vi "thorlabs_set_loopiness.vi"(8 "error in (no error)":errorcluster, 9 "PositionControlMode":i16, 10 "channel":i16, 11 "thorlabs_kinesis in":refnum<class "thorlabs_kinesis.lvclass">) -> (0 "error out":errorcluster, 3 "thorlabs_kinesis out":refnum<class "thorlabs_kinesis.lvclass">)   [LabVIEW 2015, in "thorlabs_kinesis.lvclass"]
uses:
  thorlabs_kinesis.lvclass
  thorlabs_kinesis.lvclass/thorlabs_kinesis.ctl
  thorlabs_drivers/Thorlabs.MotionControl.Benchtop.Piezo.dll
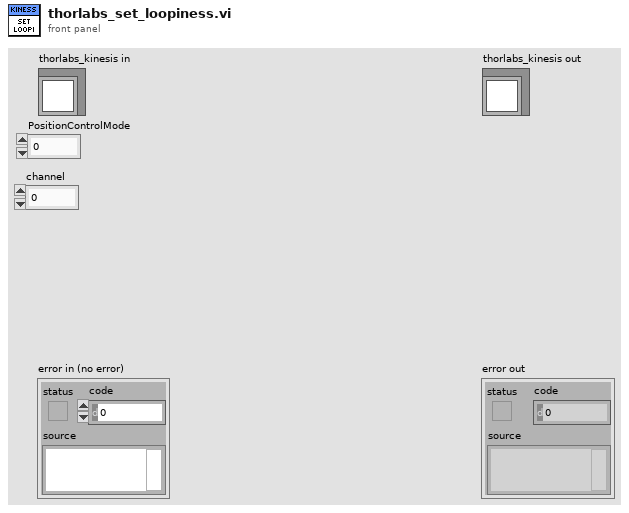
[diagram p1: front panel]
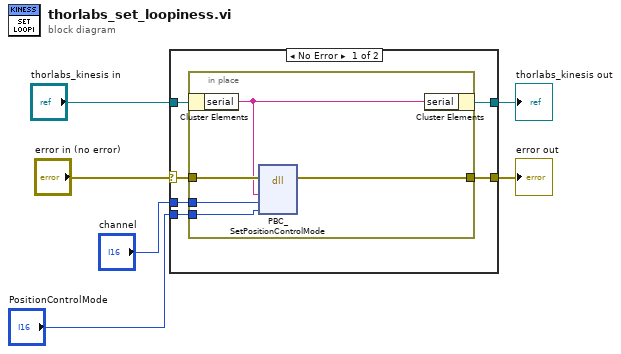
[diagram p0: block diagram]
diagram:
  n1 = case shown="No Error" "error in (no error)" {
    selector: "error in (no error)" -> [w11 w19]
    tunnel: [w10 w19] -> w5
    tunnel: [w7 w18] -> w3
    tunnel: "thorlabs_kinesis in" -> [w12 w18]
    tunnel: "PositionControlMode" -> [w9 _]
    tunnel: "channel" -> [w8 _]
    frame No Error {
      n2 = in-place {
        in-place-border: w11 -> [w17]
        in-place-border: [w16] -> w10
        in-place-border: w9 -> [w15]
        in-place-border: w8 -> [w14]
        n3 = in-place-cluster #1(w12) -> ("serial"=w13:string)
        n4 = dll-call lib="C:/Users/bspoka/Documents/LabVIEW Data/lview_180307/Stage Class/Thorlabs Kinesis/thorlabs_drivers/Thorlabs.MotionControl.Benchtop.Piezo.dll" fn="PBC_SetPositionControlMode" label="PBC_SetPositionMode"(error in=w17, "serial"=w13, "channel"=w14, "PositionControlMode"=w15) -> (error out=w16:errorcluster)  [unwired: 6 in, 1 out]
        n5 = in-place-cluster #1("serial"=w13) -> (w7:refnum<class "thorlabs_kinesis.lvclass">)
      }
    }
    frame Error {
    }
  }
  "error out" <- w5
  "thorlabs_kinesis out" <- w3
